vi "serial cmd-response.vi"(0 "VISA In":refnum<visa-resource-name>, 1 "mode":enum16{"wr & rd", "write", "read"}(ring), 3 "flush transcvr(F)":bool, 5 "cmd":string, 9 "ReadWait":u32=50, 11 "error in":errorcluster, 12 "Sem Timeout (5000)":i32=5000) -> (4 "VISA out":refnum<visa-resource-name>, 6 "rsp str out":string, 8 "cmd str out":string, 10 "timeout?":bool, 15 "error out":errorcluster)   [LabVIEW 2020]
doc: "Developed by: Kevin Thompson\nThompson Engineering\nthompson.engineering@comcast.net\n(510) 673-3614"
uses:
  <vilib>/Instr/_visa.llb/VISA Flush IO Buffer Mask.ctl
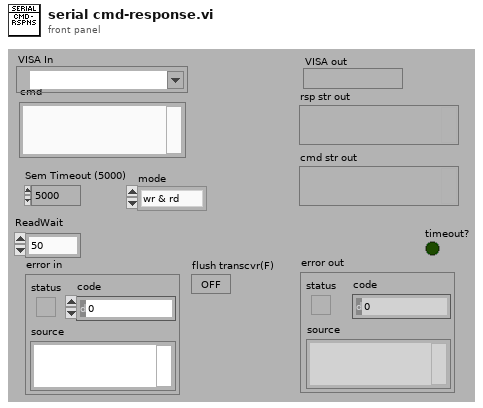
[diagram p1: front panel]
types:
  T1 = typedef "Semaphore RefNum" = refnum<k1>
  T2 = typedef "VISA Flush IO Buffer Mask.ctl" = u16
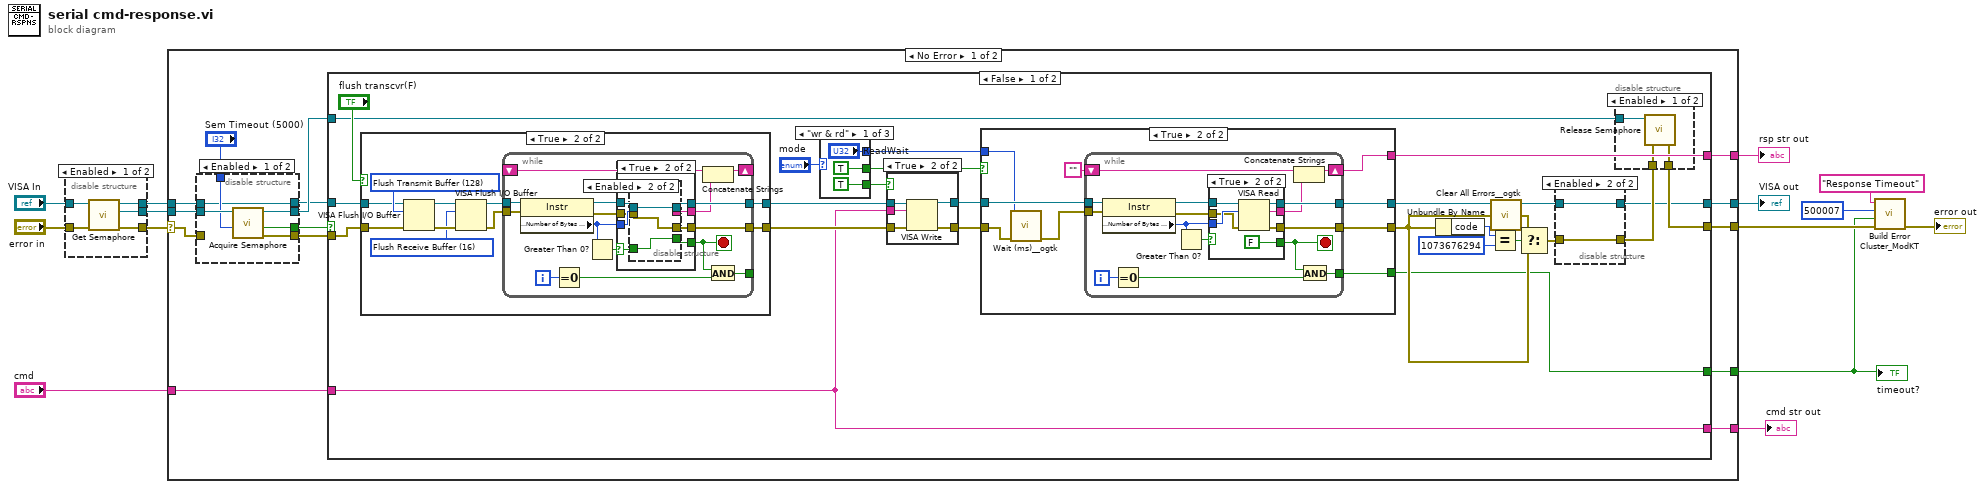
[diagram p0: block diagram]
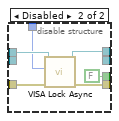
[diagram p3: hidden frame]
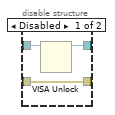
[diagram p4: hidden frame]
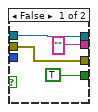
[diagram p7: hidden frame]
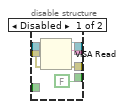
[diagram p8: hidden frame]
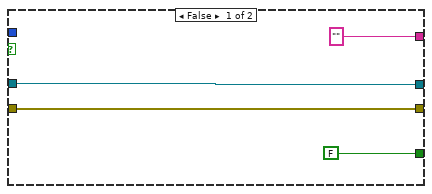
[diagram p9: hidden frame]
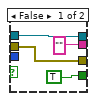
[diagram p10: hidden frame]
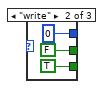
[diagram p12: hidden frame]
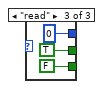
[diagram p13: hidden frame]
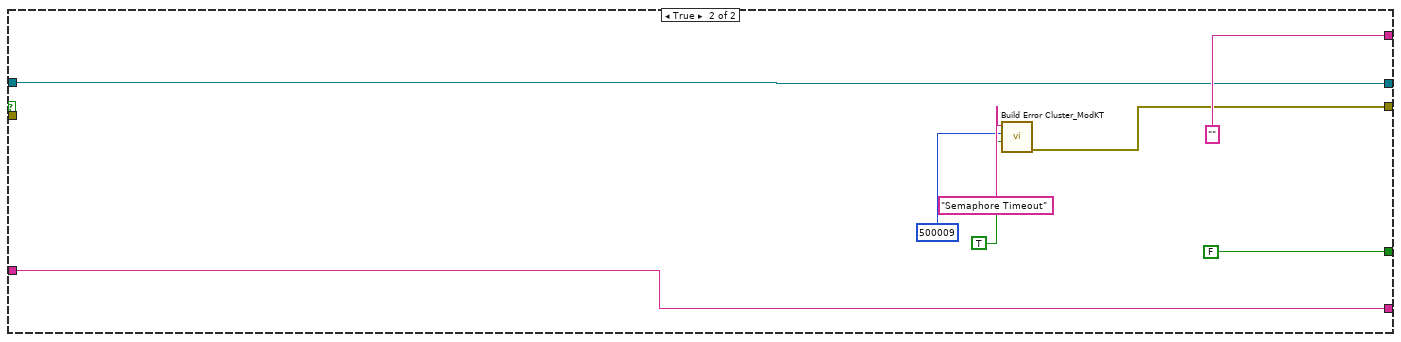
[diagram p14: hidden frame]
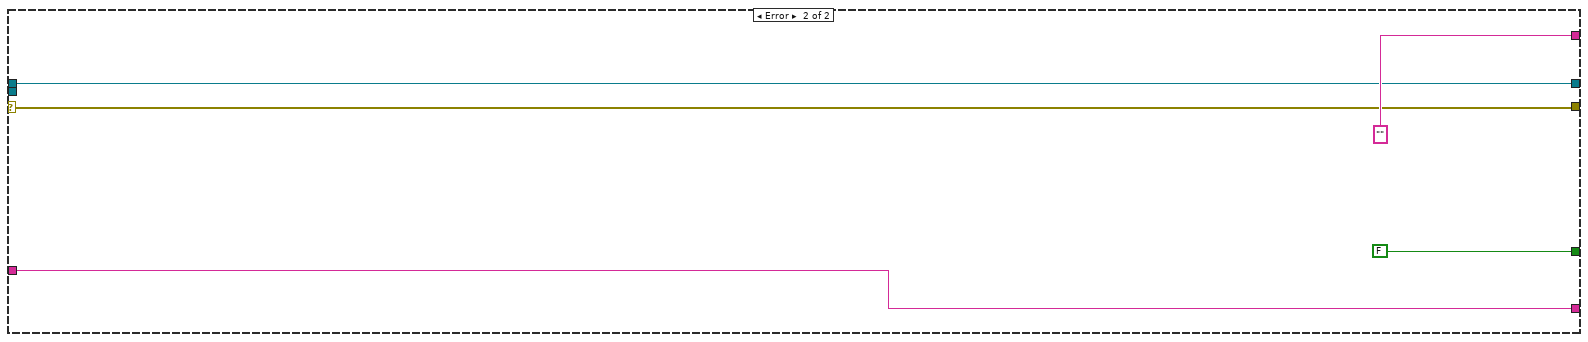
[diagram p15: hidden frame]
diagram:
  n1 = disable-structure shown="Enabled" {
    disable-tunnel: "VISA In" -> [w19 w21]
    disable-tunnel: "error in" -> [w18 w20]
    disable-tunnel: [w17 w21] -> w6
    disable-tunnel: [w16 w20] -> w5
    disable-tunnel: [w15 _] -> w4
    frame Enabled {
      n2 = call "Get Semaphore.vi"("error in"=w18, "VISA In"=w19) -> ("error out"=w16:errorcluster, "semaphore out"=w15:T1, "VISA Out"=w17:refnum<visa-resource-name>)  [unwired: 3 in]
    }
    frame Disabled {
    }
  }
  n3 = case shown="No Error" w5 {
    selector: w5 -> [w22 w195]
    tunnel: [w35 FALSE] -> w11
    tunnel: [w34 "" ("read buffer")] -> w14
    tunnel: w6 -> [w24 w196]
    tunnel: [w33 w196] -> w13
    tunnel: [w32 w195] -> w12
    tunnel: w4 -> [w31 _]
    tunnel: "cmd" -> [w26 w194]
    tunnel: [w25 w194] -> w2
    frame No Error {
      n4 = disable-structure shown="Enabled" {
        disable-tunnel: w31 -> [w41 _]
        disable-tunnel: "Sem Timeout (5000)" -> [w40 w42]
        disable-tunnel: [w39 FALSE ("timed out")] -> w29
        disable-tunnel: [w38 _] -> w28
        disable-tunnel: [w37 w47] -> w27
        disable-tunnel: w24 -> [w36 w46]
        disable-tunnel: [w36 w45] -> w23
        disable-tunnel: w22 -> [_ w44]
        frame Enabled {
          n5 = call <vilib>:"Acquire Semaphore.vi"("ms timeout (-1)"=w40, "semaphore"=w41) -> ("error out"=w37:errorcluster, "timed out"=w39:bool, "semaphore out"=w38:T1)  [unwired: 3 in]
        }
        frame Disabled {
          n6 = call <vilib>:"VISA Lock Async.vi"("error in (no error)"=w44, "timeout (0)"=w42, "VISA resource name"=w46) -> ("error out"=w47:errorcluster, "VISA resource name out"=w45:refnum<visa-resource-name>)  [unwired: 6 in, 1 out]
        }
      }
      n7 = case shown="False" w29 {
        tunnel: [w63 "" ("read buffer")] -> w34
        tunnel: [w62 FALSE] -> w35
        tunnel: w23 -> [w61 w191]
        tunnel: [w56 w188] -> w32
        tunnel: [w48 w191] -> w33
        tunnel: w28 -> [w57 _]
        tunnel: w27 -> [w55 _]
        tunnel: w26 -> [w54 w186]
        tunnel: [w54 w186] -> w25
        frame False {
          n8 = case shown="True" "flush transcvr(F)" {
            tunnel: w61 -> [w83 w92]
            tunnel: [w82 w86] -> w60
            tunnel: [w83 w87] -> w59
            tunnel: w55 -> [w82 w88]
            frame False {
            }
            frame True {
              w89 = T2 16 items=["Flush Receive Buffer"=16, "Write Transmit Buffer to Device"=32, "Flush Receive Buffer (No I/O)"=64, "Flush Transmit Buffer"=128] ("Mask")
              w93 = T2 128 items=["Flush Receive Buffer"=16, "Write Transmit Buffer to Device"=32, "Flush Receive Buffer (No I/O)"=64, "Flush Transmit Buffer"=128] ("Mask")
              n9 = VISA Flush I/O Buffer(VISA resource name=w92, mask (16)=w93, error in (no error)=w88) -> (VISA resource name out=w90:refnum<visa-resource-name>, error out=w91:errorcluster)
              n10 = VISA Flush I/O Buffer(VISA resource name=w90, mask (16)=w89, error in (no error)=w91) -> (VISA resource name out=w84:refnum<visa-resource-name>, error out=w85:errorcluster)
              n11 = while {
                tunnel: w84 -> [w108]
                tunnel: w85 -> [w103]
                tunnel: [w102] -> w87
                tunnel: [w101] -> w86
                shift-right: [w98] -> _
                shift-left: _ -> [w100]
                tunnel: [w94] -> _
                i -> [w96]
                stop <- w97 stop-if-true
                n12 = property class="Instr"(reference=w108, error in=w103) -> (reference out=w105:refnum<visa-resource-name>, error out=w106:errorcluster, "Serial Settings:Number of Bytes at Serial Port"=w104:u32)
                n13 = Equal To 0?(x=w96) -> (x = 0?=w95:bool)
                n14 = Greater Than 0?(x=w104) -> (x > 0?=w107:bool)
                n15 = case shown="True" w107 {
                  selector: w107 -> [_ w113]
                  tunnel: w104 -> [_ w120]
                  tunnel: w105 -> [w110 w114]
                  tunnel: w106 -> [w111 w119]
                  tunnel: [TRUE w118] -> w97
                  tunnel: ["" ("read buffer") w117] -> w99
                  tunnel: [w111 w116] -> w101
                  tunnel: [w110 w115] -> w102
                  frame False {
                  }
                  frame True {
                    n16 = disable-structure shown="Enabled" {
                      disable-tunnel: w120 -> [w127 _]
                      disable-tunnel: w119 -> [w126 w129]
                      disable-tunnel: [FALSE w130] -> w118
                      disable-tunnel: [w124 _] -> w117
                      disable-tunnel: [w123 w129] -> w116
                      disable-tunnel: [w122 w128] -> w115
                      disable-tunnel: w114 -> [w121 w128]
                      disable-tunnel: w113 -> [_ w130]
                      frame Disabled {
                        n17 = VISA Read(VISA resource name=w121, byte count=w127, error in (no error)=w126) -> (VISA resource name out=w122:refnum<visa-resource-name>, read buffer=w124:string, error out=w123:errorcluster)  [unwired: 1 out]
                      }
                      frame Enabled {
                      }
                    }
                  }
                }
                n18 = Concatenate Strings(w100, w99) -> (w98:string)
                n19 = And(x=w97, y=w95) -> (x .and. y?=w94:bool)
              }
            }
          }
          n20 = case shown="\"wr & rd\"" "mode" {
            tunnel: [TRUE TRUE FALSE] -> w70
            tunnel: [TRUE FALSE TRUE] -> w69
            tunnel: ["ReadWait" u32 0 ("wait (ms)") u32 0 ("wait (ms)")] -> w53
            frame "wr & rd" {
            }
            frame "write" {
            }
            frame "read" {
            }
          }
          n21 = case shown="True" w70 {
            tunnel: [w171 w176] -> w72
            tunnel: [w170 w175] -> w52
            tunnel: w59 -> [w171 w174]
            tunnel: w54 -> [_ w173]
            tunnel: w60 -> [w170 w172]
            frame False {
            }
            frame True {
              n22 = VISA Write(VISA resource name=w174, write buffer=w173, error in (no error)=w172) -> (VISA resource name out=w176:refnum<visa-resource-name>, error out=w175:errorcluster)  [unwired: 1 out]
            }
          }
          n23 = case shown="True" w69 {
            tunnel: w72 -> [w132 w143]
            tunnel: [FALSE w139] -> w62
            tunnel: [w132 w142] -> w49
            tunnel: ["" ("read buffer") w138] -> w63
            tunnel: [w131 w141] -> w64
            tunnel: w53 -> [_ w137]
            tunnel: w52 -> [w131 w136]
            frame False {
            }
            frame True {
              n24 = call <userlib>:"Wait (ms)__ogtk.vi"("error in (no error)"=w136, "milliseconds to wait"=w137) -> ("error out"=w135:errorcluster)  [unwired: 8 in, 1 out]
              n25 = while {
                tunnel: w143 -> [w158]
                tunnel: w135 -> [w153]
                tunnel: [w152] -> w142
                tunnel: [w151] -> w141
                shift-right: [w148] -> w138
                shift-left: "" -> [w150]
                tunnel: [w144] -> w139
                i -> [w146]
                stop <- w147 stop-if-true
                n26 = property class="Instr"(reference=w158, error in=w153) -> (reference out=w155:refnum<visa-resource-name>, error out=w156:errorcluster, "Serial Settings:Number of Bytes at Serial Port"=w154:u32)
                n27 = Equal To 0?(x=w146) -> (x = 0?=w145:bool)
                n28 = Greater Than 0?(x=w154) -> (x > 0?=w157:bool)
                n29 = case shown="True" w157 {
                  tunnel: w154 -> [_ w169]
                  tunnel: w155 -> [w160 w163]
                  tunnel: w156 -> [w161 w168]
                  tunnel: [TRUE FALSE] -> w147
                  tunnel: ["" ("read buffer") w166] -> w149
                  tunnel: [w161 w165] -> w151
                  tunnel: [w160 w164] -> w152
                  frame False {
                  }
                  frame True {
                    n30 = VISA Read(VISA resource name=w163, byte count=w169, error in (no error)=w168) -> (VISA resource name out=w164:refnum<visa-resource-name>, read buffer=w166:string, error out=w165:errorcluster)  [unwired: 1 out]
                  }
                }
                n31 = Concatenate Strings(w150, w149) -> (w148:string)
                n32 = And(x=w147, y=w145) -> (x .and. y?=w144:bool)
              }
            }
          }
          n33 = Unbundle By Name(w64) -> ("code"=w68:i32)
          n34 = Equal?(x=w68, y=1073676294 ("error code")) -> (x = y?=w66:bool)
          n35 = call <userlib>:"Clear All Errors__ogtk.vi"("Error In"=w64) -> ("Error Out"=w65:errorcluster)  [unwired: 3 in]
          n36 = Select(t=w65, s=w66, f=w64) -> (s? t:f=w51:errorcluster)
          n37 = disable-structure shown="Enabled" {
            disable-tunnel: w51 -> [w73 w76]
            disable-tunnel: [w73 w76] -> w50
            disable-tunnel: w49 -> [w75 w77]
            disable-tunnel: [w74 w77] -> w48
            frame Disabled {
              n38 = VISA Unlock(11:w75) -> (3:w74:refnum<visa-resource-name>)  [unwired: 1 in, 1 out]
            }
            frame Enabled {
            }
          }
          n39 = disable-structure shown="Enabled" {
            disable-tunnel: w57 -> [w80 _]
            disable-tunnel: w50 -> [w79 w81]
            disable-tunnel: [w78 w81] -> w56
            frame Enabled {
              n40 = call <vilib>:"Release Semaphore.vi"("error in (no error)"=w79, "semaphore"=w80) -> ("error out"=w78:errorcluster)  [unwired: 4 in, 1 out]
            }
            frame Disabled {
            }
          }
        }
        frame True {
          n41 = call <vilib>:"Build Error Cluster_ModKT .vi"("Prepend String (\"\")"="Semaphore Timeout" ("Prepend String (\"\")"), "code"=500009, "error? (F)"=TRUE) -> ("error out"=w188:errorcluster)  [unwired: 4 in, 1 out]
        }
      }
    }
    frame Error {
    }
  }
  "timeout?" <- w11
  "rsp str out" <- w14
  "VISA out" <- w13
  "cmd str out" <- w2
  n42 = call <vilib>:"Build Error Cluster_ModKT .vi"("Prepend String (\"\")"="Response Timeout" ("Prepend String (\"\")"), "code"=500007, "error? (F)"=w11, "error in (no error)"=w12) -> ("error out"=→"error out":errorcluster)  [unwired: 3 in, 1 out]
